vi "MGCC_Version2_MGCC_FntStaMach_Visualization_OpalRT_HTBnoBatt.vi"() -> ()   [LabVIEW 2016]
panel:
  in  "PV Mode":bool
  out "Communication 3":bool
  out "Active power control":bool
  out "Reactive power control":bool
  out "Output":dbl format="%#_4f"
  out "Communication 2":bool
  out "Resynchronization":bool
  out "Active power control 2":bool
  out "Reactive power control 2":bool
  out "SOC":dbl format="%#_4f"
  out "Output 2":dbl format="%#_4f"
  out "W3":bool
  out "I 8":dbl format="%#.4f"
  out "I 7":dbl format="%#.4f"
  out "I 6":dbl format="%#.4f"
  out "I 5":dbl format="%#.4f"
  out "I 4":dbl format="%#.4f"
  out "I 3":dbl format="%#.4f"
  out "I 2":dbl format="%#.4f"
  out "I 1":dbl format="%#.4f"
  out "Current State":string
  out "Model Mgmt.":bool
  out "PV Forecasting":bool
  out "Load Forecasting":bool
  out "PQ Balance":bool
  out "Black Start":bool
  out "Data Logging":bool
  out "Communication":bool
  out "State Estimation":bool
  out "Energy Mgmt.":bool
  out "L4":cluster{dbl[], dbl[]}(graph)
  out "L8":cluster{dbl[], dbl[]}(graph)
  out "L6":cluster{dbl[], dbl[]}(graph)
  out "B1":cluster{dbl[], dbl[]}(graph)
  out "PV":cluster{dbl[], dbl[]}(graph)
  out "L7":cluster{dbl[], dbl[]}(graph)
  out "L3":cluster{dbl[], dbl[]}(graph)
  out "G2":cluster{dbl[], dbl[]}(graph)
  out "L2":cluster{dbl[], dbl[]}(graph)
  out "L1":cluster{dbl[], dbl[]}(graph)
  out "G1":cluster{dbl[], dbl[]}(graph)
  in  "Stop":bool
  in  "RESET":bool
  in  "G2":bool
  in  "G1":bool
  in  "Ready for STD":bool
  in  "Recon cmd":bool
  in  "BKS cmd":bool
  in  "island cmd":bool
  out "PV Forecast":dbl[](graph)
  out "Sources Power":T1(graph)
  out "Frequency":T2(graph)
  in  "Power Tabs":T3(tab)
  out "Loads Power":dbl(graph)
  out "Loads Power 2":dbl(graph)
  out "Loads Power 3":dbl(graph)
  out "Loads Power 4":dbl(graph)
  out "Loads Power 5":dbl(graph)
  out "Loads Power 6":dbl(graph)
  out "Loads Power 7":dbl(graph)
  out "Loads Power 8":dbl(graph)
  in  "Voltage Tabs":T3(tab)
  out "Voltage":dbl(graph)
  out "Voltage 2":dbl(graph)
  out "Voltage 3":dbl(graph)
  out "Voltage 4":dbl(graph)
  out "Voltage 5":dbl(graph)
  out "Voltage 6":dbl(graph)
  out "Voltage 7":dbl(graph)
  out "Voltage 8":dbl(graph)
  out "L4":bool
  out "L8":bool
  out "L6":bool
  out "B1":bool
  out "Bess1 Slider":dbl(slide) scale=0.0..1.0
  out "PV":bool
  out "L7":bool
  out "W9":bool
  out "I6":bool
  out "W5":bool
  out "I7":bool
  out "W6":bool
  out "I8":bool
  out "W7":bool
  out "I5":bool
  out "I4":bool
  out "W4":bool
  out "I3":bool
  out "W8":bool
  out "I2":bool
  out "W2":bool
  out "I1":bool
  out "W1":bool
  out "L3":bool
  out "G2":bool
  out "L2":bool
  out "L1":bool
  out "G1":bool
  # "Hardware Test Bed Controller"
  # "Central Controller"
  # "G2"
  # "L3"
  # "G1"
  # "L1"
  # "L2"
  # "BESS1"
  # "PV"
  # "L6"
  # "L7"
  # "L8"
  # "L4"
  # "PV Local Controller"
  # "Battery Local Controller"
  # "-Manual"
  # "-Profile"
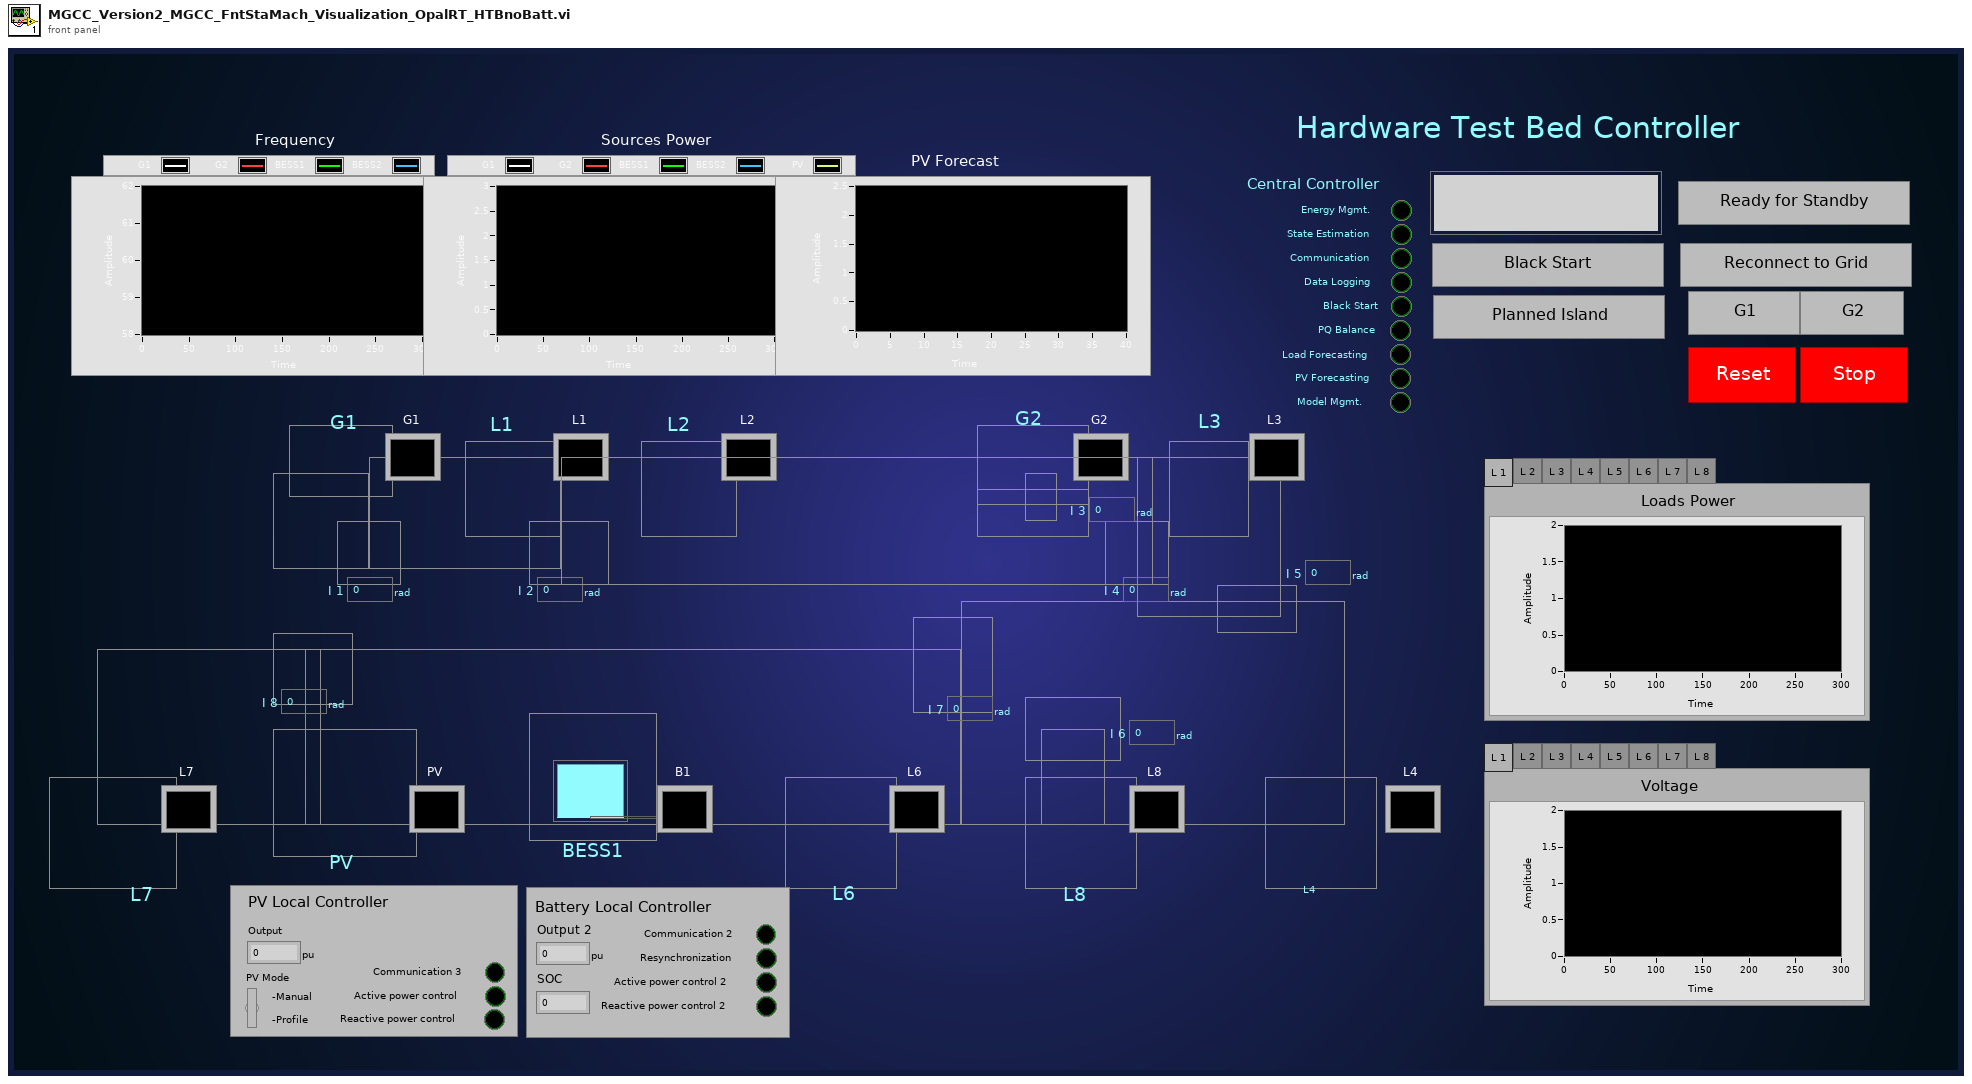
[diagram p1: front panel]
types:
  T1 = cluster{"Double":dbl, "Double":dbl, "Double":dbl, "Double":dbl, "Double":dbl}
  T2 = cluster{"Double":dbl, "Double":dbl, "Double":dbl, "Double":dbl}
  T3 = enum32{"L 1", "L 2", "L 3", "L 4", "L 5", "L 6", "L 7", "L 8"}
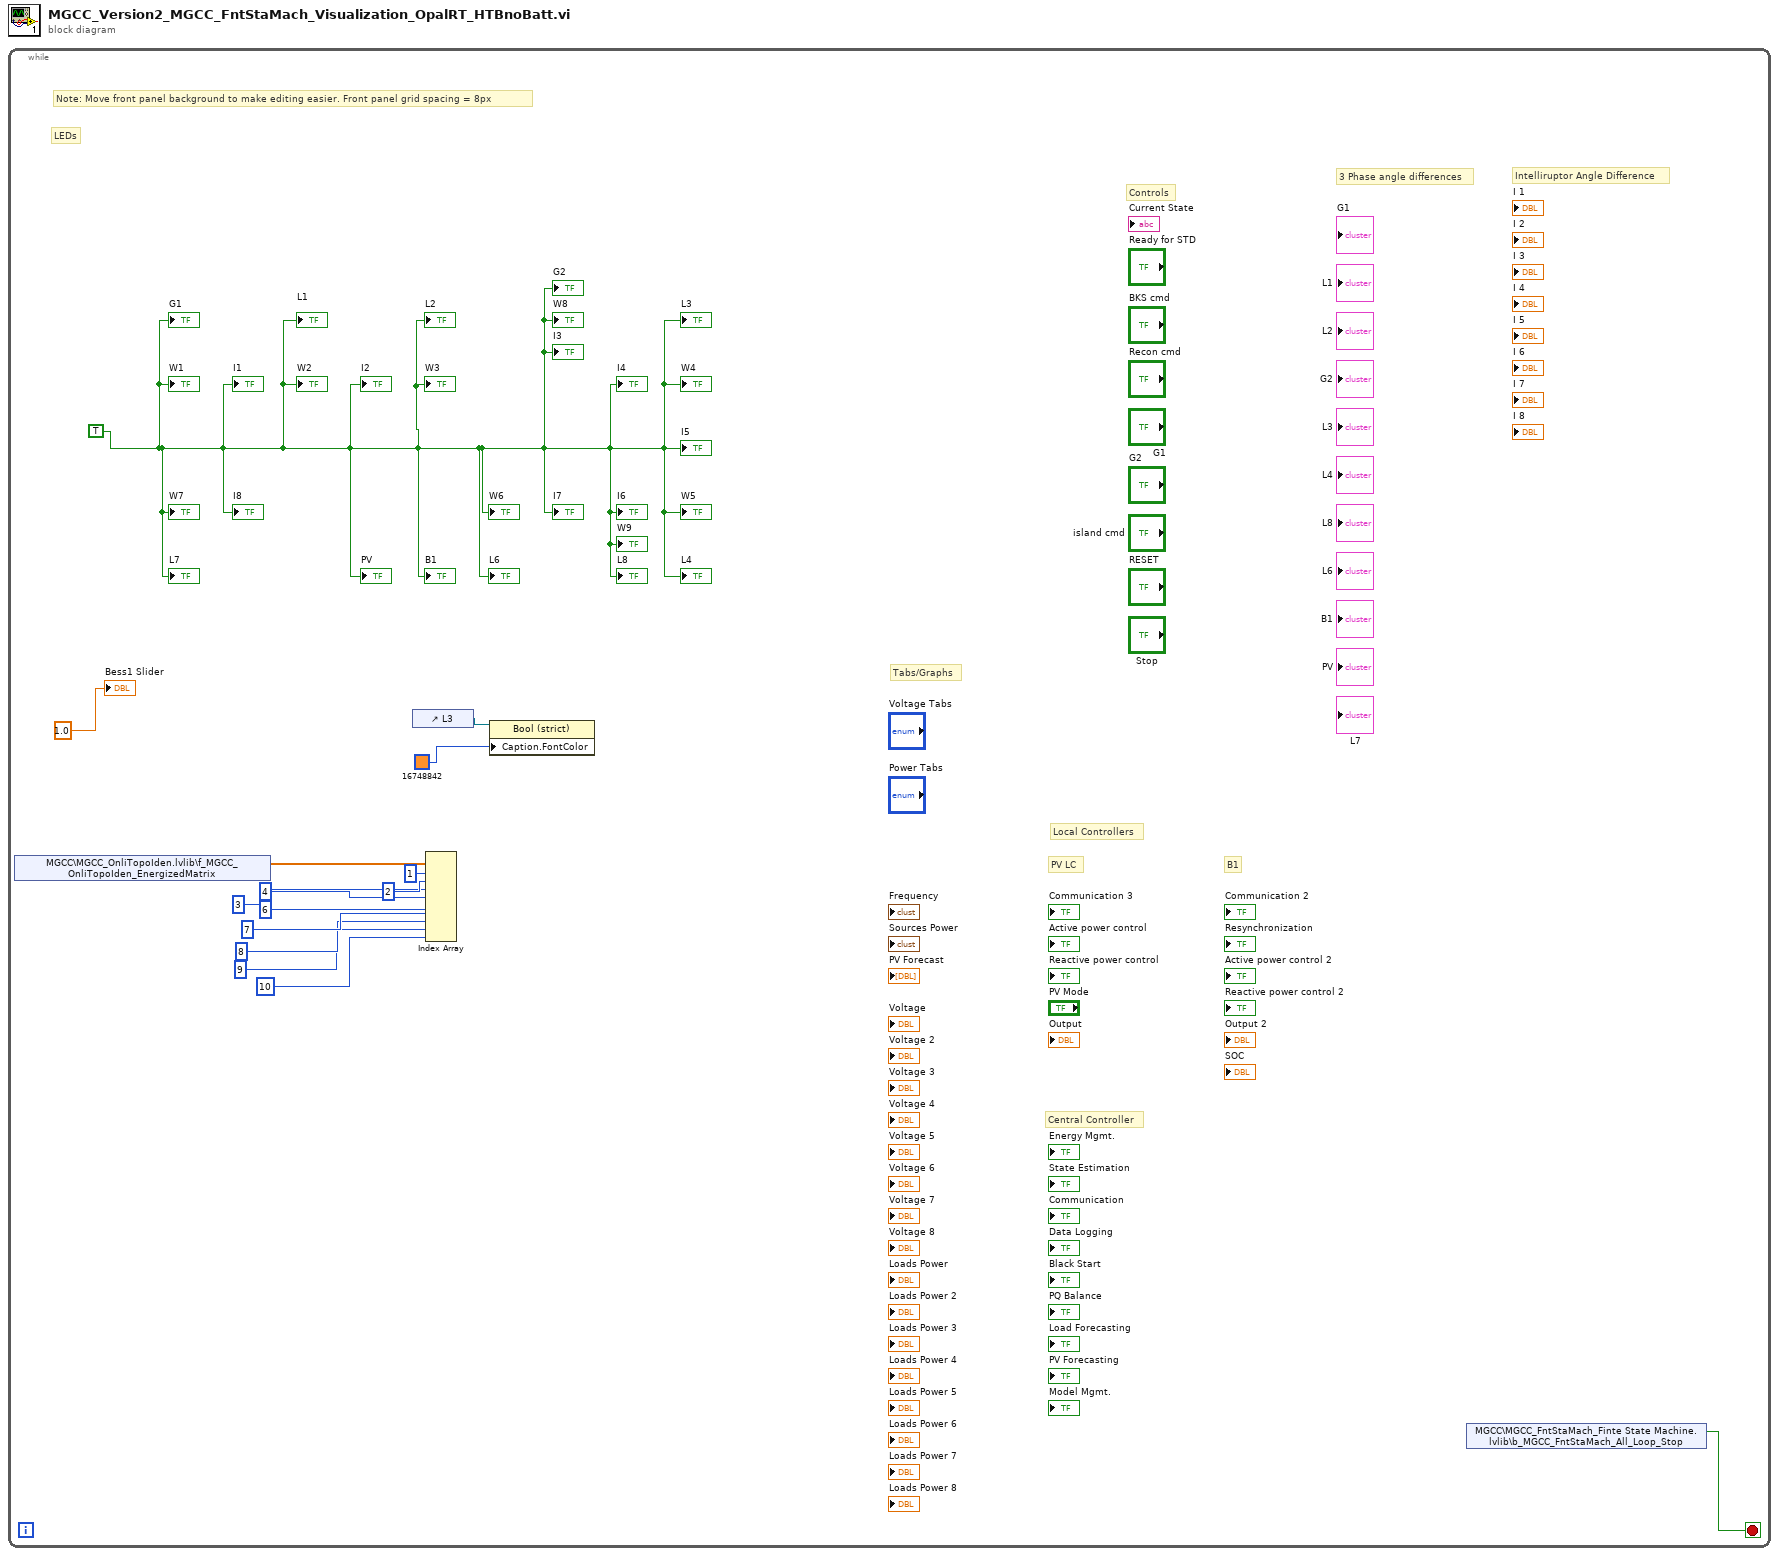
[diagram p0: block diagram]
diagram:
  n1 = while {
    stop <- w11 stop-if-true
    w14 = TRUE
    # "Note: Move front panel background to make editing easier. Front panel grid spacing = 8px"
    # "Intelliruptor Angle Difference"
    # "B1"
    # "Central Controller"
    # "Local Controllers"
    # "PV LC"
    # "3 Phase angle differences"
    # "Controls"
    # "Tabs/Graphs"
    # "LEDs"
    n2 = shared-variable "MGCC\\MGCC_OnliTopoIden.lvlib\\f_MGCC_OnliTopoIden_EnergizedMatrix"() -> (w10:dbl[])  [unwired: 1 in, 1 out]
    n3 = control-ref of="L3"() -> (w13:refnum<vi>)
    n4 = Index Array(array=w10, index #1=1 ("index"), index #2=2 ("index"), index #3=3 ("index"), index #4=4 ("index"), index #5=6 ("index"), index #6=7 ("index"), index #7=8 ("index"), index #8=9 ("index"), index #9=10 ("index")) -> ()  [unwired: 9 out]
    n5 = property on="Property Node" class="Bool (strict)"(reference=w13, "Caption.FontColor"=u32 16748842) -> ()  [unwired: 1 in, 2 out]
    n6 = shared-variable "MGCC\\MGCC_FntStaMach_Finte State Machine.lvlib\\b_MGCC_FntStaMach_All_Loop_Stop"() -> (w11:bool)  [unwired: 1 in, 1 out]
    "G1" <- w14
    "L1" <- w14
    "L2" <- w14
    "G2" <- w14
    "L3" <- w14
    "W1" <- w14
    "I1" <- w14
    "W2" <- w14
    "I2" <- w14
    "W8" <- w14
    "I3" <- w14
    "I4" <- w14
    "W4" <- w14
    "I5" <- w14
    "W7" <- w14
    "I8" <- w14
    "W6" <- w14
    "I7" <- w14
    "W5" <- w14
    "I6" <- w14
    "W9" <- w14
    "L7" <- w14
    "PV" <- w14
    "B1" <- w14
    "L6" <- w14
    "L8" <- w14
    "L4" <- w14
    "Bess1 Slider" <- 1.0 ("Slide 2")
    "W3" <- w14
  }
